vi "Write With Delay.vi"(6 "Delay Time (s)":dbl=0.1, 8 "error in":errorcluster, 10 "write buffer":string, 11 "VISA resource name":refnum<visa-resource-name>) -> (0 "error out":errorcluster, 3 "VISA resource name out":refnum<visa-resource-name>)   [LabVIEW 2019, in "Acopian.lvlib" / "Acopian.lvclass"]
uses:
  Library/Acopian.lvclass
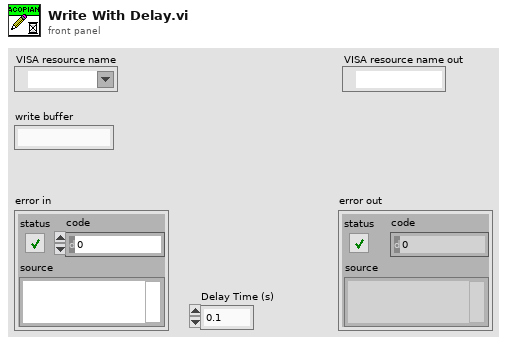
[diagram p1: front panel]
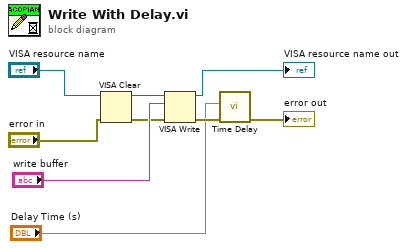
[diagram p0: block diagram]
diagram:
  n1 = VISA Clear(VISA resource name="VISA resource name", error in (no error)="error in") -> (VISA resource name out=w4:refnum<visa-resource-name>, error out=w2:errorcluster)
  n2 = VISA Write(VISA resource name=w4, write buffer="write buffer", error in (no error)=w2) -> (VISA resource name out=→"VISA resource name out":refnum<visa-resource-name>, error out=w7:errorcluster)  [unwired: 1 out]
  n3 = call "Time Delay"("error in (no error)"=w7, "Delay Time (s)"="Delay Time (s)") -> ("error out"=→"error out":errorcluster)  [unwired: 9 in]
